vi "HCC Cycle Count Checker.vi"(0 "Input Cycle Count":u16, 1 "Total Cycle Count (Current)":u16, 5 "Error In":errorcluster) -> (14 "Input Cycle Count OUT":u16, 15 "Total Cycle Count (Current) OUT":u16, 16 "Enter Timer Loop":bool, 17 "Reset Timer":bool, 18 "Timer Limit":dbl, 19 "Error Out":errorcluster)   [LabVIEW 2016]
uses:
  Type Definitions/HCC Cycle Check Conditions.ctl
panel:
  out "Conditions":T1
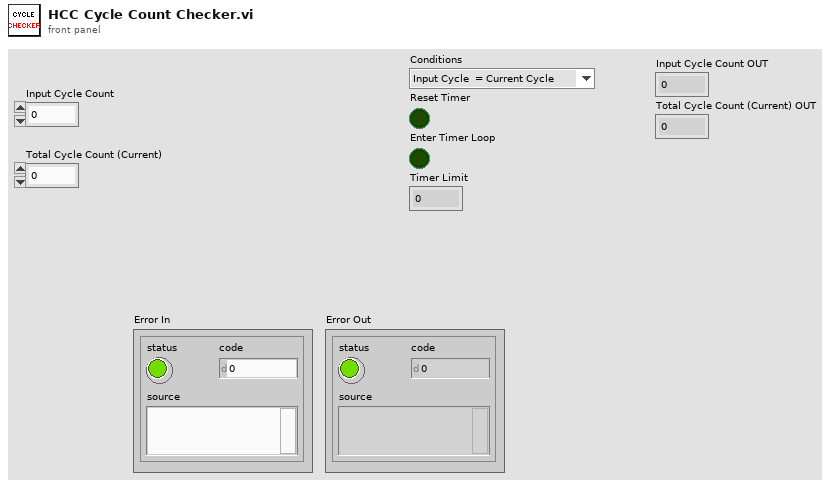
[diagram p1: front panel]
types:
  T1 = typedef "HCC Cycle Check Conditions.ctl" = enum16{"Input Cycle  = Current Cycle", "Input Cycle = 1-Current Cycle", "Input Cycle = 1+Current Cycle", "Input Cycle = <1-Current Cycle", "Input Cycle = >1+Current Cycle"}
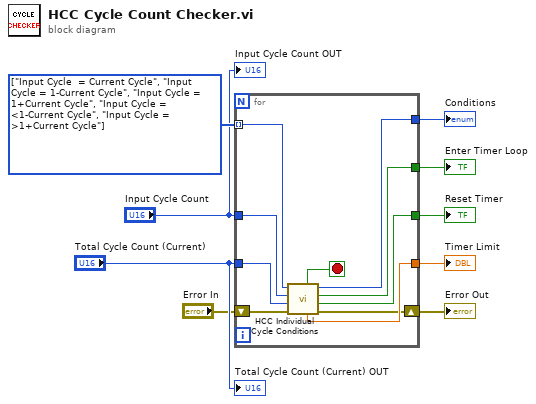
[diagram p0: block diagram]
diagram:
  w9 = T1[] [enum."Input Cycle  = Current Cycle", enum."Input Cycle = 1-Current Cycle", enum."Input Cycle = 1+Current Cycle", enum."Input Cycle = <1-Current Cycle", enum."Input Cycle = >1+Current Cycle"] items=["Input Cycle  = Current Cycle", "Input Cycle = 1-Current Cycle", "Input Cycle = 1+Current Cycle", "Input Cycle = <1-Current Cycle", "Input Cycle = >1+Current Cycle"]
  n1 = for {
    tunnel: w9 -> [w19] mode=indexing
    tunnel: "Input Cycle Count" -> [w18]
    tunnel: "Total Cycle Count (Current)" -> [w17]
    tunnel: [w15] -> w3
    tunnel: [w14] -> w6
    tunnel: [w13] -> w5
    tunnel: [w12] -> w4
    shift-right: [w10] -> w1
    shift-left: "Error In" -> [w11]
    stop <- w16 stop-if-true
    n2 = call "HCC Individual Cycle Conditions.vi"("Error In"=w11, "Total Cycle Count (Current)"=w17, "Input Cycle Count"=w18, "Conditions in"=w19) -> ("Error Out"=w10:errorcluster, "Reset Timer"=w13:bool, "Enter Timer Loop"=w14:bool, "Conditions out"=w15:T1, "Timer Limit"=w12:dbl, "Stop Loop"=w16:bool)  [unwired: 2 in]
  }
  "Reset Timer" <- w5
  "Enter Timer Loop" <- w6
  "Timer Limit" <- w4
  "Conditions" <- w3
  "Error Out" <- w1
  "Input Cycle Count OUT" <- "Input Cycle Count"
  "Total Cycle Count (Current) OUT" <- "Total Cycle Count (Current)"
